vi "Corr Transducers Load INFO.vi"(7 "item ref":refnum<vi>, 8 "error in":errorcluster, 11 "Path":path) -> (0 "error out":errorcluster, 3 "transducer info":T1)   [LabVIEW 2020]
doc: "Transducer correction INFO loader."
uses:
  Corr Transducer INFO Record.ctl
  Corr Transducer INFO Item.ctl
  Corr CSV Template.ctl
  octave/infolib/GetString.vi
  <vilib>/Utility/error.llb/Error Cluster From Error Code.vi
  octave/infolib/GetEXT.vi
  <vilib>/ErrorRing/Error Ring.xnode
  octave/infolib/infolib.lvlib
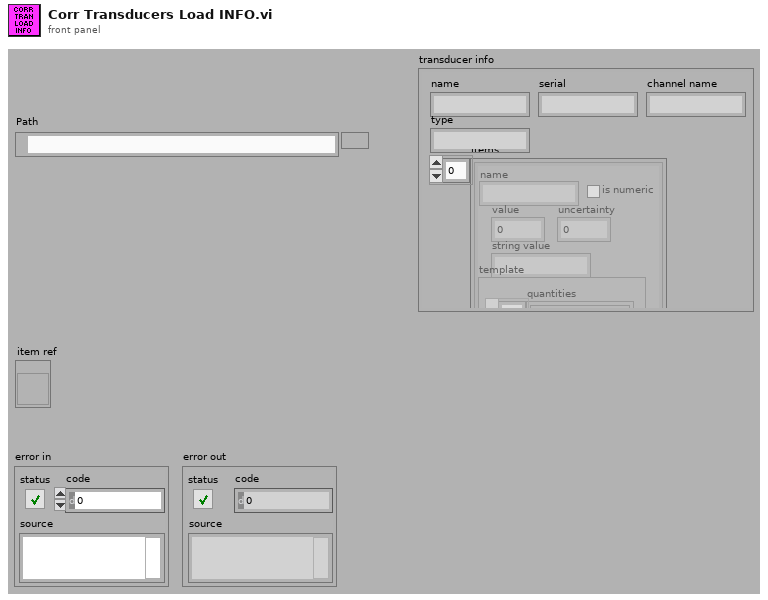
[diagram p1: front panel]
types:
  T1 = typedef "Corr Transducer INFO Record.ctl" = cluster{"name":string, "serial":string, "channel name":string, "items":T2[], "type":string}
  T2 = typedef "Corr Transducer INFO Item.ctl" = cluster{"name":string, "is numeric":bool, "value":dbl, "uncertainty":dbl, "string value":string, "template":T3, "info":string}
  T3 = typedef "Corr CSV Template.ctl" = cluster{"quantities":string[], "y-axis":string, "x-axis":string}
  T4 = cluster{"name":string, "numeric":bool, "template":T3, "info":string}[]
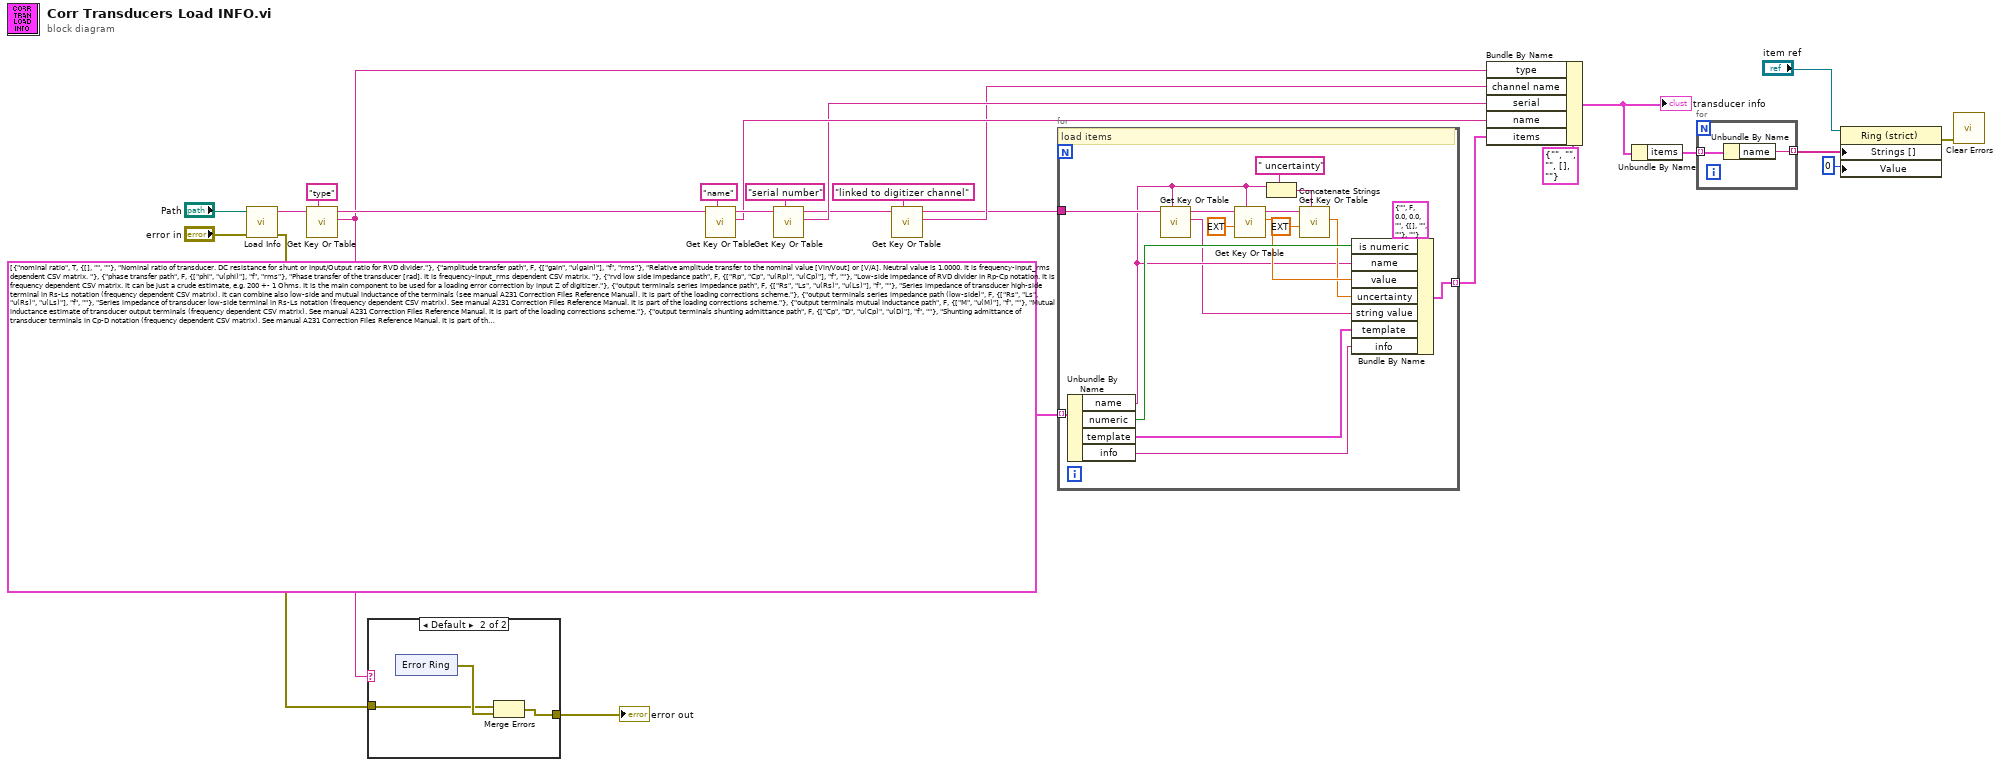
[diagram p0: block diagram]
diagram:
  n1 = call "Load Info.vi"("error in"="error in", "filename"="Path") -> ("error out"=w2:errorcluster, "info data"=w24:string)  [unwired: 8 in]
  n2 = call-poly "Get Key Or Table.vi"("key description"="type", "info data"=w24) -> ("value"=w3:string, "info data out"=w22:string)  [unwired: 6 in, 2 out]
  n3 = case shown="Default" w3 {
    tunnel: w2 -> [w27 w29]
    tunnel: [w27 w28] -> w1
    frame "divider", "shunt" {
    }
    frame Default {
      n4 = xnode "Error Ring"() -> ("error out"=w30:errorcluster)
      n5 = Merge Errors(w29, w30) -> (w28:errorcluster)
    }
  }
  "error out" <- w1
  n6 = call-poly "Get Key Or Table.vi"("key description"="name", "info data"=w22) -> ("value"=w10:string, "info data out"=w13:string)  [unwired: 6 in, 2 out]
  n7 = call-poly "Get Key Or Table.vi"("key description"="serial number", "info data"=w13) -> ("value"=w9:string, "info data out"=w7:string)  [unwired: 6 in, 2 out]
  n8 = call-poly "Get Key Or Table.vi"("key description"="linked to digitizer channel", "info data"=w7) -> ("value"=w5:string, "info data out"=w4:string)  [unwired: 6 in, 2 out]
  n9 = for {
    tunnel: T4 [{"name"="nominal ratio", "numeric"=TRUE, "template"={"quantities"=[], "y-axis"="", "x-axis"=""}, "info"="Nominal ratio of transducer. DC resistance for shunt or Input/Output ratio for RVD divider."}, {"name"="amplitude transfer path", "numeric"=FALSE, "template"={"quantities"=["gain", "u(gain)"], "y-axis"="f", "x-axis"="rms"}, "info"="Relative amplitude transfer to the nominal value [Vin/Vout] or [V/A]. Neutral value is 1.0000. It is frequency-input_rms dependent CSV matrix. "}, {"name"="phase transfer path", "numeric"=FALSE, "template"={"quantities"=["phi", "u(phi)"], "y-axis"="f", "x-axis"="rms"}, "info"="Phase transfer of the transducer [rad]. It is frequency-input_rms dependent CSV matrix. "}, {"name"="rvd low side impedance path", "numeric"=FALSE, "template"={"quantities"=["Rp", "Cp", "u(Rp)", "u(Cp)"], "y-axis"="f", "x-axis"=""}, "info"="Low-side impedance of RVD divider in Rp-Cp notation. It is frequency dependent CSV matrix. It can be just a crude estimate, e.g. 200 +- 1 Ohms. It is the main component to be used for a loading error correction by input Z of digitizer."}, {"name"="output terminals series impedance path", "numeric"=FALSE, "template"={"quantities"=["Rs", "Ls", "u(Rs)", "u(Ls)"], "y-axis"="f", "x-axis"=""}, "info"="Series impedance of transducer high-side terminal in Rs-Ls notation (frequency dependent CSV matrix). It can combine also low-side and mutual inductance of the terminals (see manual A231 Correction Files Reference Manual). It is part of the loading corrections scheme."}, {"name"="output terminals series impedance path (low-side)", "numeric"=FALSE, "template"={"quantities"=["Rs", "Ls", "u(Rs)", "u(Ls)"], "y-axis"="f", "x-axis"=""}, "info"="Series impedance of transducer low-side terminal in Rs-Ls notation (frequency dependent CSV matrix). See manual A231 Correction Files Reference Manual. It is part of the loading corrections scheme."}, {"name"="output terminals mutual inductance path", "numeric"=FALSE, "template"={"quantities"=["M", "u(M)"], "y-axis"="f", "x-axis"=""}, "info"="Mutual inductance estimate of transducer output terminals (frequency dependent CSV matrix). See manual A231 Correction Files Reference Manual. It is part of the loading corrections scheme."}, {"name"="output terminals shunting admittance path", "numeric"=FALSE, "template"={"quantities"=["Cp", "D", "u(Cp)", "u(D)"], "y-axis"="f", "x-axis"=""}, "info"="Shunting admittance of transducer terminals in Cp-D notation (frequency dependent CSV matrix). See manual A231 Correction Files Reference Manual. It is part of the loading corrections scheme."}, {"name"="output cable series impedance path", "numeric"=FALSE, "template"={"quantities"=["Rs", "Ls", "u(Rs)", "u(Ls)"], "y-axis"="f", "x-axis"=""}, "info"="Series impedance of output cable in Rs-Ls notation (frequency dependent CSV matrix). See manual A231 Correction Files Reference Manual. It is part of the loading corrections scheme."}, {"name"="output cable shunting admittance path", "numeric"=FALSE, "template"={"quantities"=["Cp", "D", "u(Cp)", "u(D)"], "y-axis"="f", "x-axis"=""}, "info"="Shunting admittance of output cable in Cp-D notation (frequency dependent CSV matrix). See manual A231 Correction Files Reference Manual. It is part of the loading corrections scheme."}, {"name"="buffer output series impedance path", "numeric"=FALSE, "template"={"quantities"=["Rs", "Ls", "u(Rs)", "u(Ls)"], "y-axis"="f", "x-axis"=""}, "info"="Eventual series impedance of a buffer placed between transduce output and cable in Rs-Ls notation (frequency dependent CSV matrix). See manual A231 Correction Files Reference Manual. It is part of the loading corrections scheme."}, {"name"="sfdr path", "numeric"=FALSE, "template"={"quantities"=["sfdr"], "y-axis"="f", "x-axis"="a"}, "info"="SFDR value of the transducer (frequency-amplitude dependent CSV matrix). It is used for estimation of harmonics and THD uncertainty and positive values are expected, e.g. +105 dBc means harmonics are at least 105 dB lower than carrier."}] -> [w52] mode=indexing
    tunnel: w4 -> [w42]
    tunnel: [w39] -> w6 mode=indexing
    # "load items"
    n10 = Unbundle By Name(w52) -> ("name"=w41:string, "numeric"=w51:bool, "template"=w37:T3, "info"=w36:string)
    n11 = call-poly "Get Key Or Table.vi"("key description"=w41, "info data"=w42) -> ("value"=w40:string, "info data out"=w43:string)  [unwired: 6 in, 2 out]
    n12 = call-poly "Get Key Or Table.vi"("key description"=w41, "numeric"=ext 1.0, "info data"=w43) -> ("value"=w45:ext, "info data out"=w49:string)  [unwired: 5 in, 2 out]
    n13 = Concatenate Strings(w41, " uncertainty" ("string")) -> (w47:string)
    n14 = call-poly "Get Key Or Table.vi"("key description"=w47, "numeric"=ext 0.0, "info data"=w49) -> ("value"=w44:ext)  [unwired: 5 in, 3 out]
    n15 = Bundle By Name(cluster=T2 {"name"="", "is numeric"=FALSE, "value"=0.0, "uncertainty"=0.0, "string value"="", "template"={"quantities"=[], "y-axis"="", "x-axis"=""}, "info"=""} ("transducer item"), "is numeric"=w51, "name"=w41, "value"=w45, "uncertainty"=w44, "string value"=w40, "template"=w37, "info"=w36) -> (w39:T2)
  }
  n16 = Bundle By Name(cluster=T1 {"name"="", "serial"="", "channel name"="", "items"=[], "type"=""} ("transducer info"), "type"=w3, "channel name"=w5, "serial"=w9, "name"=w10, "items"=w6) -> (w21:T1)
  "transducer info" <- w21
  n17 = Unbundle By Name(w21) -> ("items"=w20:T2[])
  n18 = for {
    tunnel: w20 -> [w54] mode=indexing
    tunnel: [w53] -> w18 mode=indexing
    n19 = Unbundle By Name(w54) -> ("name"=w53:string)
  }
  n20 = property class="Ring (strict)"(reference="item ref", "Strings []"=w18, "Value"=u16 0) -> (error out=w16:errorcluster)  [unwired: 1 in, 1 out]
  n21 = call <vilib>:"Clear Errors.vi"("error in (no error)"=w16) -> ()  [unwired: 5 in, 2 out]
